vi "RFID_connection.vi"(9 "Estado_de_conexion":bool, 10 "Puerto RFID":u16, 11 "IP RFID":string) -> (2 "RFID_connection_text":string, 3 "RFID connection":bool)   [LabVIEW 2015]
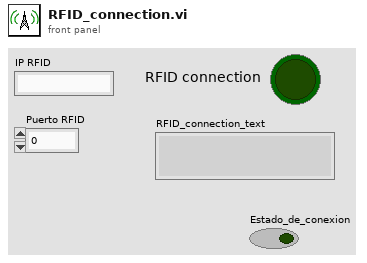
[diagram p1: front panel]
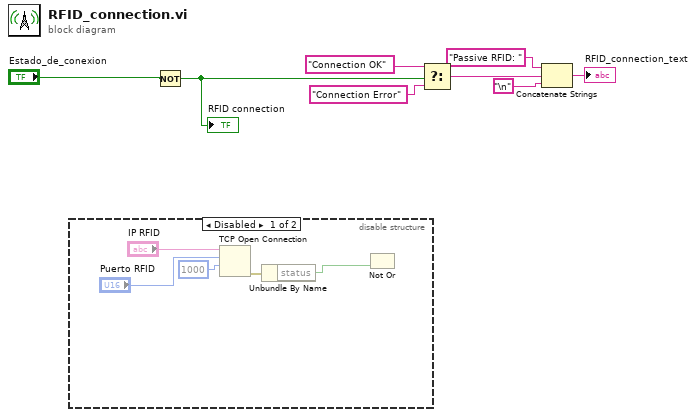
[diagram p0: block diagram]
diagram:
  n1 = disable-structure shown="Disabled" {
    frame Disabled {
      n2 = TCP Open Connection(address="IP RFID", remote port or service name="Puerto RFID", timeout ms (60000)=1000) -> (error out=w13:errorcluster)  [unwired: 2 in, 1 out]
      n3 = Unbundle By Name(w13) -> ("status"=w9:bool)
      n4 = Not Or(1:w9) -> ()  [unwired: 1 in, 1 out]
    }
    frame Enabled {
    }
  }
  n5 = Not(x="Estado_de_conexion") -> (.not. x?=w1:bool)
  "RFID connection" <- w1
  n6 = Select(t="Connection OK" ("string"), s=w1, f="Connection Error") -> (s? t:f=w6:string)
  n7 = Concatenate Strings("Passive RFID: " ("string"), w6, "\n") -> (→"RFID_connection_text":string)
